vi "Lookup Device.vi"(8 "error in (no error)":errorcluster, 10 "Type":string, 11 "HAL Manager in":refnum<class "HAL Manager.lvclass">) -> (0 "error out":errorcluster, 2 "Device":refnum<class "Device.lvclass">, 3 "HAL Manager out":refnum<class "HAL Manager.lvclass">)   [LabVIEW 2020, in "HAL.lvlib" / "HAL Manager.lvclass"]
uses:
  HAL Manager.lvclass
  Device/Device.lvclass
  HAL Manager.lvclass/HAL Manager.ctl
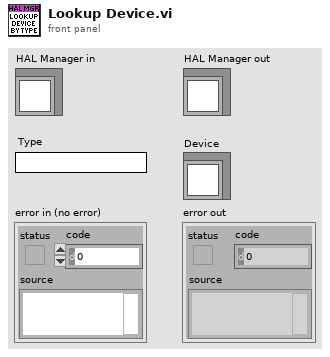
[diagram p1: front panel]
types:
  T1 = typedef "HAL.lvlib/HAL Manager.lvclass/Ref Data.ctl" = cluster{"Devices":refnum<class "Device.lvclass">[], "Type":string[], "Models":string[], "Name":string[]}
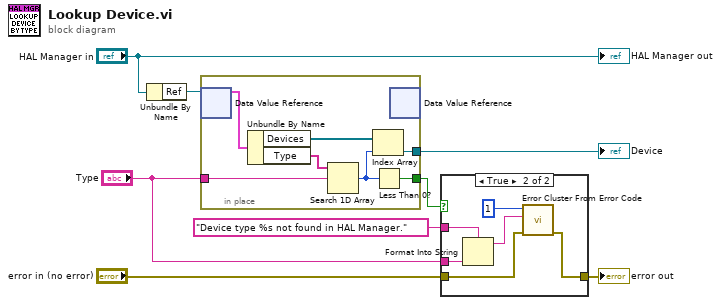
[diagram p0: block diagram]
diagram:
  n1 = Unbundle By Name("HAL Manager in") -> ("Ref"=w8:refnum<data-value>)
  n2 = in-place {
    in-place-border: "Type" -> [w14]
    in-place-border: [w11] -> w6
    in-place-border: [w9] -> w4
    n3 = in-place-dvr #1(w8) -> (w15:T1)  [unwired: 1 out]
    n4 = Unbundle By Name(w15) -> ("Devices"=w12:refnum<class "Device.lvclass">[], "Type"=w13:string[])
    n5 = Search 1D Array(1D array=w13, element=w14) -> (index of element=w10:i32)  [unwired: 1 in]
    n6 = Index Array(array=w12, index=w10) -> (element=w11:refnum<class "Device.lvclass">)
    n7 = Less Than 0?(x=w10) -> (x < 0?=w9:bool)
    n8 = in-place-dvr #1() -> ()  [unwired: 1 in, 2 out]
  }
  "Device" <- w6
  n9 = case shown="True" w4 {
    tunnel: "error in (no error)" -> [w16 w22]
    tunnel: [w16 w20] -> w3
    tunnel: "Type" -> [_ w18]
    tunnel: "Device type %s not found in HAL Manager." -> [_ w19]
    frame False {
    }
    frame True {
      n10 = Format Into String(format string=w19, w18) -> (resulting string=w17:string)  [unwired: 2 in, 1 out]
      n11 = call <vilib>:"Error Cluster From Error Code.vi"("error in (no error)"=w22, "error message (\"\")"=w17, "error code (0)"=1) -> ("error out"=w20:errorcluster)  [unwired: 6 in]
    }
  }
  "error out" <- w3
  "HAL Manager out" <- "HAL Manager in"
